vi "MW测试.vi"() -> ()   [LabVIEW 2016]
panel:
  out "数值":sgl format="%_6g"
  in  "数值类型":enum16{"长整型", "双精度"}(ring)
  in  "值 2":sgl format="%.3g"
  in  "TCP操作模式":enum16{"打开TCP", "读MW区", "写MW区", "关闭TCP"}(ring)
  in  "布尔":bool
  in  "TCP连接参数":cluster{"IP地址":string, "端口":u16}={"IP地址"="192.168.1.88", "端口"=502}
  in  "值":i32=10
  in  "寄存器MD地址":i32=10
  out "值":u32
  out "x-y":u32
  out "读写OK":bool
  in  "停止":bool
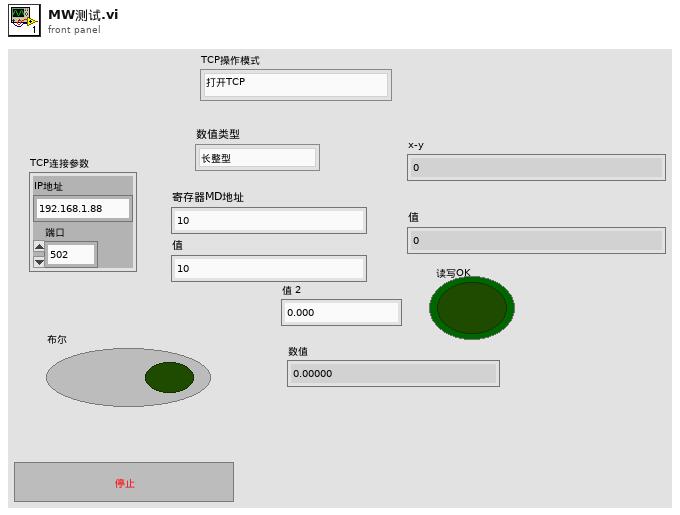
[diagram p1: front panel]
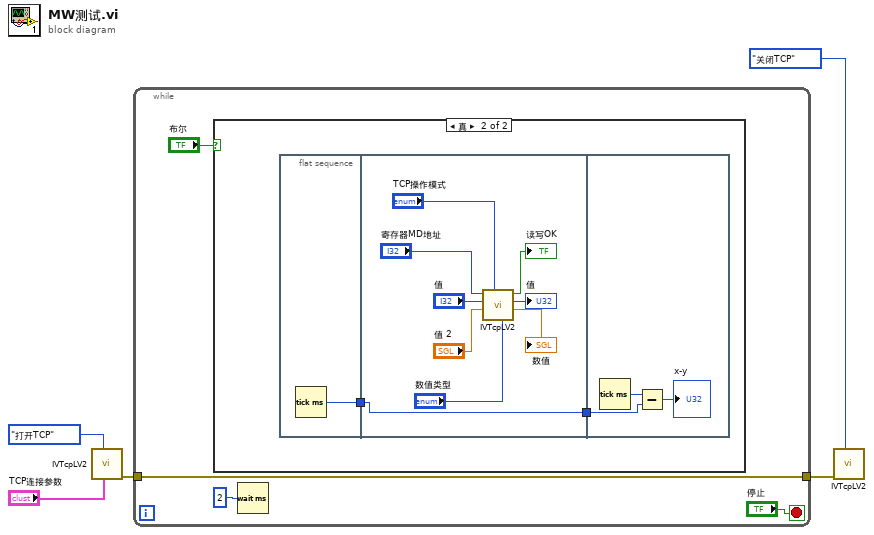
[diagram p0: block diagram]
diagram:
  n1 = call "IVTcpLV2.vi"("TCP连接参数"="TCP连接参数", "TCP操作模式"=enum16{"打开TCP", "读MW区", "写MW区", "关闭TCP"}."打开TCP") -> ("错误输出"=w3:errorcluster)  [unwired: 6 in, 3 out]
  n2 = while {
    tunnel: w3 -> [w7]
    tunnel: [w7] -> w1
    stop <- "停止" stop-if-true
    n3 = case shown="真" "布尔" {
      frame False {
      }
      frame True {
        n4 = flat-sequence {
          tunnel: [w12] -> w11
          tunnel: [w20] -> w10
          tunnel: w11 -> [w20]
          tunnel: w10 -> [w23]
          frame #0 {
            n5 = Tick Count (ms)() -> (millisecond timer value=w12:u32)
          }
          frame #1 {
            n6 = call "IVTcpLV2.vi"("数值类型"="数值类型", "TCP操作模式"="TCP操作模式", 9:"值"="值 2", 10:"值"="值", "寄存器MD地址"="寄存器MD地址") -> (1:"数值"=→"数值":sgl, 2:"数值"=→"值":u32, "=1？"=→"读写OK":bool)  [unwired: 3 in, 1 out]
          }
          frame #2 {
            n7 = Tick Count (ms)() -> (millisecond timer value=w24:u32)
            n8 = Subtract(x=w24, y=w23) -> (x-y=→"x-y":u32)
          }
        }
      }
    }
    n9 = Wait (ms)(milliseconds to wait=u32 2 ("等待时间（毫秒）")) -> ()  [unwired: 1 out]
  }
  n10 = call "IVTcpLV2.vi"("TCP操作模式"=enum16{"打开TCP", "读MW区", "写MW区", "关闭TCP"}."关闭TCP", "错误输入"=w1) -> ()  [unwired: 6 in, 4 out]
